vi "Write With Abort.vi"(6 "abort":bool, 10 "element":cluster{timestamp[], dbl[]}[](array[cluster])) -> (2 "channel":T1, 4 "aborted?":bool, 5 "previous element":cluster{timestamp[], dbl[]}[](array[cluster]))   [LabVIEW 2020, in "Tag-a[.](c(a[.](stamp),a[.](dbl))).lvlib"]
doc: "Writes a value to a Tag channel or signals the channel to abort. This endpoint is the same as the Write endpoint except that it has an <B>abort</B> input and an <B>aborted?</B> output. You can use the abort capability of the Tag channel to close a channel abruptly, ignoring any data left in the channel buffer. You must use this endpoint together with the Read With Abort endpoint."
uses:
  <extravilib>/ChannelInstances/Tag-a[.](c(a[.](stamp),a[.](dbl))).lvlib
  <extravilib>/ChannelInstances/Tag-a[.](c(a[.](stamp),a[.](dbl)))/))Channel.ctl
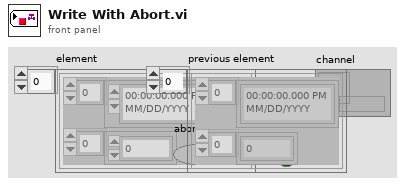
[diagram p1: front panel]
types:
  T1 = typedef "Tag-a[.](c(a[.](stamp),a[.](dbl))).lvlib/))Channel.ctl" = refnum<queue>
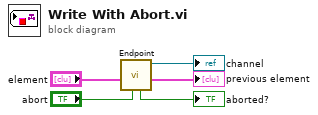
[diagram p0: block diagram]
diagram:
  n1 = call <extravilib>:"Endpoint.vi"("abort (F)"="abort", "element in"="element") -> ("element out"=→"previous element":cluster{timestamp[], dbl[]}[], "channel out"=→"channel":T1, "aborted?"=→"aborted?":bool)  [unwired: 6 in, 1 out]
